vi "DeInit.vi"(8 "error in (no error)":errorcluster, 11 "PLCHandler in":refnum<class "PLCHandler.lvclass">) -> (0 "error out":errorcluster, 3 "PLCHandler out":refnum<class "PLCHandler.lvclass">)   [LabVIEW 2022 SP3, in "PLCHandler.lvlib" / "PLCHandler.lvclass"]
uses:
  PLCHandler.lvclass
  PLCHandler.lvclass/PLCHandler.ctl
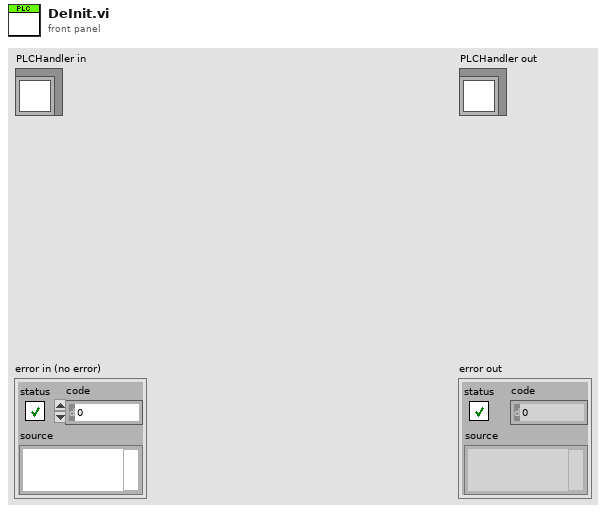
[diagram p1: front panel]
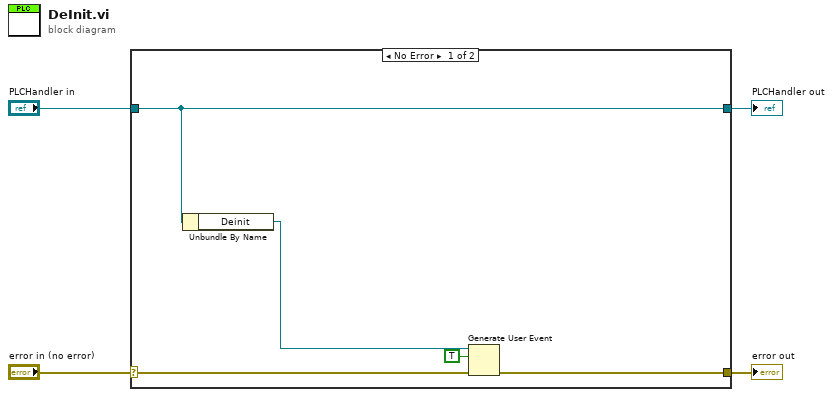
[diagram p0: block diagram]
diagram:
  n1 = case shown="No Error" "error in (no error)" {
    selector: "error in (no error)" -> [w9 w11]
    tunnel: [w8 w11] -> w3
    tunnel: [w7 w10] -> w1
    tunnel: "PLCHandler in" -> [w7 w10]
    frame No Error {
      n2 = Unbundle By Name(w7) -> ("Deinit"=w6:refnum<user-event>)
      n3 = Generate User Event(user event=w6, event data cluster=TRUE ("event data"), error in=w9) -> (error out=w8:errorcluster)  [unwired: 1 in, 1 out]
    }
    frame Error {
    }
  }
  "error out" <- w3
  "PLCHandler out" <- w1
